vi "new file extension.vi"(1 "new extension":string, 2 "input path":path) -> (0 "output path&filename":path)   [LabVIEW 2022 SP3]
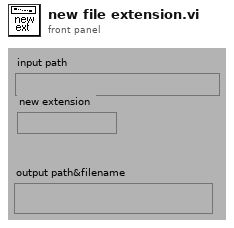
[diagram p1: front panel]
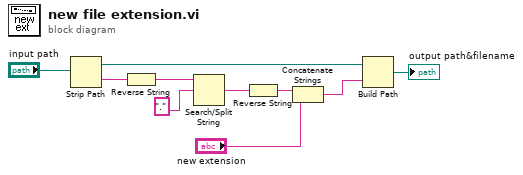
[diagram p0: block diagram]
diagram:
  n1 = Strip Path(path="input path") -> (stripped path=w8:path, name=w5:string)
  n2 = Reverse String(1:w5) -> (0:w4:string)
  n3 = Search/Split String(string=w4, search string/char (-)=".") -> (match + rest of string=w3:string)  [unwired: 1 in, 2 out]
  n4 = Reverse String(1:w3) -> (0:w2:string)
  n5 = Concatenate Strings(w2, "new extension") -> (w9:string)
  n6 = Build Path(base path=w8, name or relative path=w9) -> (appended path=→"output path&filename":path)
